vi "setting.vi"() -> ()   [LabVIEW 2019, in "Setting Lib.lvlib"]
uses:
  Setting Lib.lvlib
  User Lib.lvlib
  Calibration Lib.lvlib
  database.lvlib
panel:
  out "Error out 4":errorcluster
  in  "Error in 2":errorcluster
  out "Error out 3":errorcluster
  out "Error out 2":errorcluster
  out "Error out":errorcluster
  out "String":string
  in  "Close":bool
  in  "Calibration":bool
  in  "General":bool
  in  "Speed Control":bool
  in  "User":bool
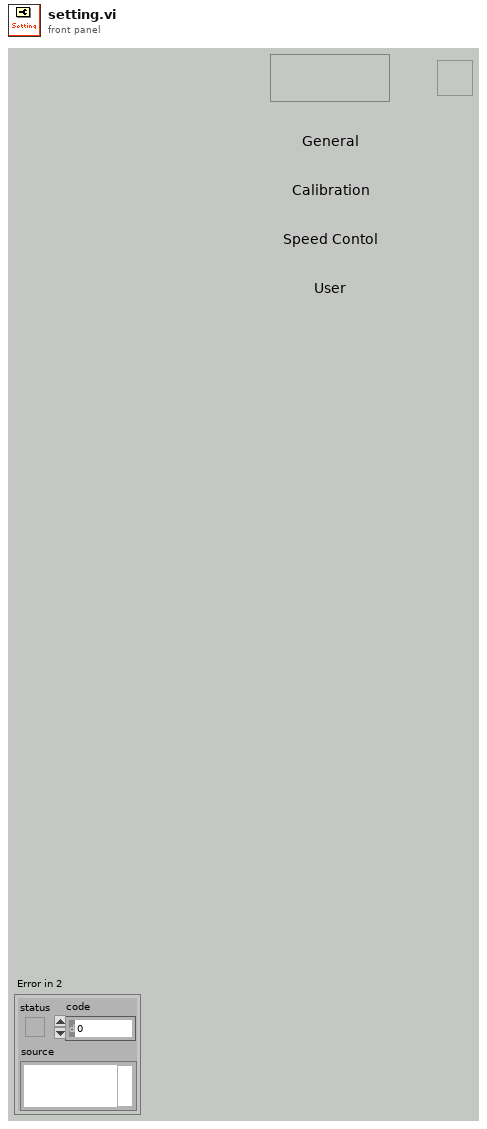
[diagram p1: front panel]
types:
  T1 = cluster{string, "date/time string":string, "date/time string":string, string}
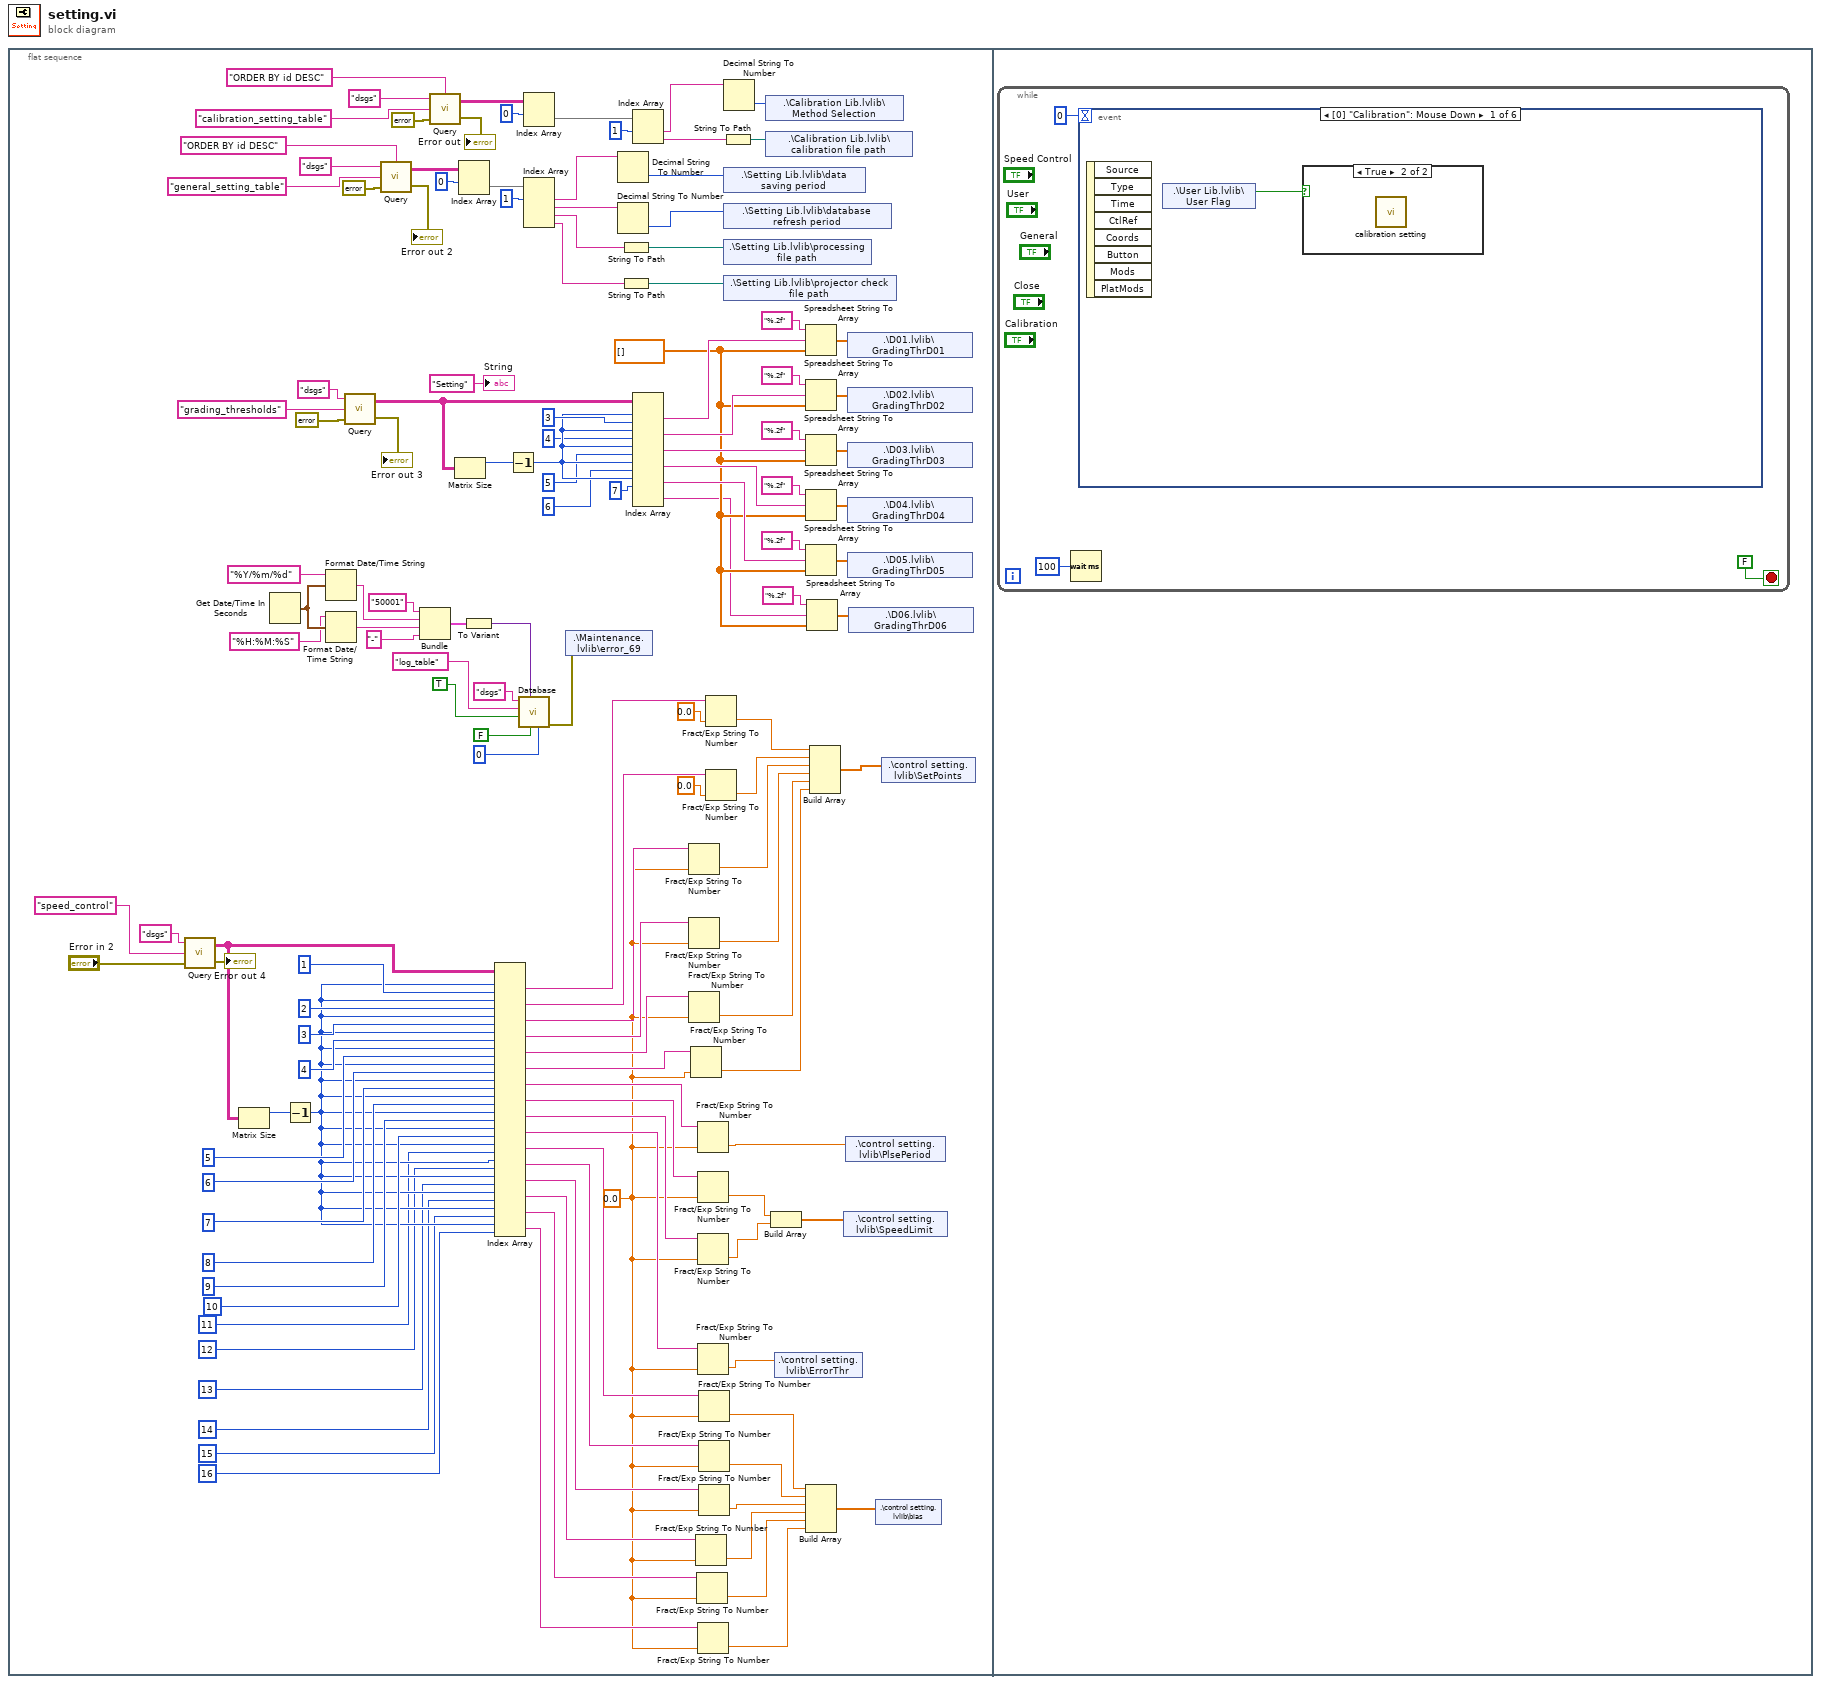
[diagram p0: block diagram]
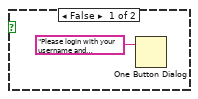
[diagram p2: hidden frame]
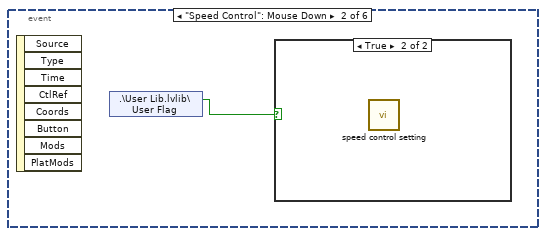
[diagram p3: hidden frame]
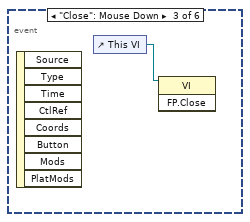
[diagram p5: hidden frame]
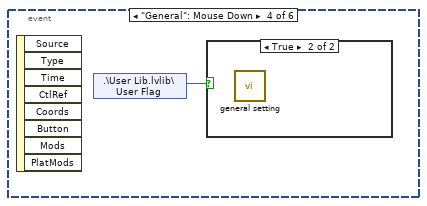
[diagram p6: hidden frame]
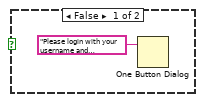
[diagram p7: hidden frame]
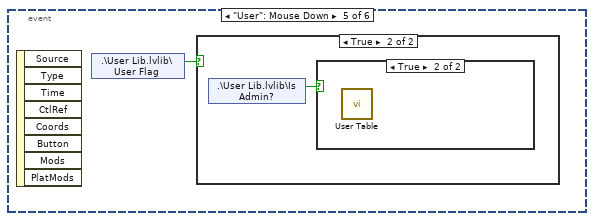
[diagram p8: hidden frame]
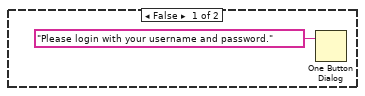
[diagram p9: hidden frame]
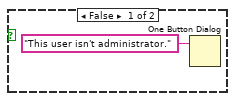
[diagram p10: hidden frame]
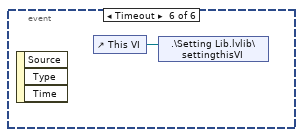
[diagram p11: hidden frame]
diagram:
  n1 = flat-sequence {
    frame #0 {
      w8 = 0.0 ("default (0 DBL)")
      w30 = dbl[] []
      n2 = call "Query.vi"("Error in"="Error in 2", "Table Name"="speed_control", "Connection Name"="dsgs") -> ("Error out"=→"Error out 4":errorcluster, "data"=w45:string[][])  [unwired: 1 in]
      n3 = Matrix Size(0:w45) -> (1:w62:i32)  [unwired: 1 out]
      n4 = Get Date/Time In Seconds() -> (seconds since 1Jan1904=w77:timestamp)
      n5 = Decrement(x=w62) -> (x-1=w21:i32)
      n6 = Format Date/Time String(time format string (%c)="%Y/%m/%d", seconds (now)=w77) -> (date/time string=w74:string)  [unwired: 1 in]
      n7 = Format Date/Time String(time format string (%c)="%H:%M:%S", seconds (now)=w77) -> (date/time string=w73:string)  [unwired: 1 in]
      n8 = call "Query.vi"("Error in"=errorcluster {"status"=FALSE, "code"=0, "source"=""}, "Table Name"="grading_thresholds", "Connection Name"="dsgs") -> ("Error out"=→"Error out 3":errorcluster, "data"=w136:string[][])  [unwired: 1 in]
      n9 = call "Query.vi"("Condition"="ORDER BY id DESC", "Error in"=errorcluster {"status"=FALSE, "code"=0, "source"=""}, "Table Name"="general_setting_table", "Connection Name"="dsgs") -> ("Error out"=→"Error out 2":errorcluster, "data"=w108:string[][])
      n10 = Bundle("50001", "date/time string"=w74, "date/time string"=w73, "-") -> (w71:T1)  [unwired: 1 in]
      n11 = call "Query.vi"("Condition"="ORDER BY id DESC", "Error in"=errorcluster {"status"=FALSE, "code"=0, "source"=""}, "Table Name"="calibration_setting_table", "Connection Name"="dsgs") -> ("Error out"=→"Error out":errorcluster, "data"=w90:string[][])
      n12 = Matrix Size(0:w136) -> (1:w135:i32)  [unwired: 1 out]
      n13 = Index Array(array=w108, index (row)=0) -> (element=w106:string[])  [unwired: 1 in]
      n14 = To Variant(anything=w71) -> (Variant=w70:variant)
      n15 = Index Array(array=w45, index (row) #1=w21, index (col) #1=1 ("disabled index (col)"), index (row) #2=w21, index (col) #2=2 ("disabled index (col)"), index (row) #3=w21, index (col) #3=3 ("disabled index (col)"), index (row) #4=w21, index (col) #4=4 ("disabled index (col)"), index (row) #5=w21, index (col) #5=5 ("disabled index (col)"), index (row) #6=w21, index (col) #6=6 ("disabled index (col)"), index (row) #7=w21, index (col) #7=7 ("disabled index (col)"), index (row) #8=w21, index (col) #8=8 ("disabled index (col)"), index (row) #9=w21, index (col) #9=9 ("disabled index (col)"), index (row) #10=w21, index (col) #10=10 ("disabled index (col)"), index (row) #11=w21, index (col) #11=11 ("disabled index (col)"), index (row) #12=w21, index (col) #12=12 ("disabled index (col)"), index (row) #13=w21, index (col) #13=13 ("disabled index (col)"), index (row) #14=w21, index (col) #14=14 ("disabled index (col)"), index (row) #15=w21, index (col) #15=15 ("disabled index (col)"), index (row) #16=w21, index (col) #16=16 ("disabled index (col)")) -> (element #1=w52:string, element #2=w49:string, element #3=w48:string, element #4=w47:string, element #5=w46:string, element #6=w23:string, element #7=w24:string, element #8=w25:string, element #9=w26:string, element #10=w27:string, element #11=w14:string, element #12=w13:string, element #13=w12:string, element #14=w11:string, element #15=w10:string, element #16=w9:string)
      n16 = Decrement(x=w135) -> (x-1=w133:i32)
      n17 = call "Database.vi"("Maximum Row"=u64 0 ("Storage Time (Day)"), "Delete row?"=FALSE, "Data"=w70, "Auto Increment ID?"=TRUE, "Table"="log_table", "Connection"="dsgs") -> ("Error out"=w66:errorcluster)  [unwired: 5 in]
      n18 = Index Array(array=w90, index (row)=0) -> (element=w92:string[])  [unwired: 1 in]
      n19 = Index Array(array=w106, index #1=1 ("index")) -> (element #1=w104:string, element #2=w103:string, element #3=w102:string, element #4=w101:string)  [unwired: 3 in]
      n20 = shared-variable ".\\Maintenance.lvlib\\error_69"(w66) -> ()  [unwired: 1 in, 1 out]
      n21 = Decimal String To Number(string=w104) -> (number=w97:i32)  [unwired: 2 in, 1 out]
      n22 = Decimal String To Number(string=w103) -> (number=w98:i32)  [unwired: 2 in, 1 out]
      n23 = String To Path(string=w102) -> (path=w99:path)
      n24 = String To Path(string=w101) -> (path=w100:path)
      n25 = Index Array(array=w92, index #1=1 ("index")) -> (element #1=w94:string, element #2=w85:string)  [unwired: 1 in]
      n26 = Index Array(array=w136, index (row) #1=w133, index (col) #1=3 ("disabled index (col)"), index (row) #2=w133, index (col) #2=4 ("disabled index (col)"), index (row) #3=w133, index (col) #3=5 ("disabled index (col)"), index (row) #4=w133, index (col) #4=6 ("disabled index (col)"), index (row) #5=w133, index (col) #5=7 ("disabled index (col)")) -> (element #1=w128:string, element #2=w122:string, element #3=w121:string, element #4=w120:string, element #5=w119:string, element #6=w29:string)  [unwired: 2 in]
      n27 = Fract/Exp String To Number(string=w48, default (0 dbl)=w8) -> (number=w42:dbl)  [unwired: 2 in, 1 out]
      n28 = Fract/Exp String To Number(string=w47, default (0 dbl)=w8) -> (number=w41:dbl)  [unwired: 2 in, 1 out]
      n29 = Fract/Exp String To Number(string=w46, default (0 dbl)=w8) -> (number=w40:dbl)  [unwired: 2 in, 1 out]
      n30 = Fract/Exp String To Number(string=w23, default (0 dbl)=w8) -> (number=w22:dbl)  [unwired: 2 in, 1 out]
      n31 = Fract/Exp String To Number(string=w11, default (0 dbl)=w8) -> (number=w4:dbl)  [unwired: 2 in, 1 out]
      n32 = Fract/Exp String To Number(string=w10, default (0 dbl)=w8) -> (number=w3:dbl)  [unwired: 2 in, 1 out]
      n33 = Fract/Exp String To Number(string=w24, default (0 dbl)=w8) -> (number=w38:dbl)  [unwired: 2 in, 1 out]
      n34 = Fract/Exp String To Number(string=w25, default (0 dbl)=w8) -> (number=w37:dbl)  [unwired: 2 in, 1 out]
      n35 = Fract/Exp String To Number(string=w26, default (0 dbl)=w8) -> (number=w36:dbl)  [unwired: 2 in, 1 out]
      n36 = Fract/Exp String To Number(string=w27, default (0 dbl)=w8) -> (number=w34:dbl)  [unwired: 2 in, 1 out]
      n37 = Fract/Exp String To Number(string=w9, default (0 dbl)=w8) -> (number=w2:dbl)  [unwired: 2 in, 1 out]
      n38 = Fract/Exp String To Number(string=w14, default (0 dbl)=w8) -> (number=w7:dbl)  [unwired: 2 in, 1 out]
      n39 = Fract/Exp String To Number(string=w13, default (0 dbl)=w8) -> (number=w6:dbl)  [unwired: 2 in, 1 out]
      n40 = Fract/Exp String To Number(string=w12, default (0 dbl)=w8) -> (number=w5:dbl)  [unwired: 2 in, 1 out]
      n41 = Fract/Exp String To Number(string=w52, default (0 dbl)=0.0 ("default (0 DBL)")) -> (number=w44:dbl)  [unwired: 2 in, 1 out]
      n42 = Fract/Exp String To Number(string=w49, default (0 dbl)=0.0 ("default (0 DBL)")) -> (number=w43:dbl)  [unwired: 2 in, 1 out]
      n43 = String To Path(string=w85) -> (path=w95:path)
      n44 = Decimal String To Number(string=w94) -> (number=w96:i32)  [unwired: 2 in, 1 out]
      n45 = shared-variable ".\\Setting Lib.lvlib\\data saving period"(w97) -> ()  [unwired: 1 in, 1 out]
      n46 = shared-variable ".\\Setting Lib.lvlib\\database refresh period"(w98) -> ()  [unwired: 1 in, 1 out]
      n47 = shared-variable ".\\Setting Lib.lvlib\\processing file path"(w99) -> ()  [unwired: 1 in, 1 out]
      n48 = shared-variable ".\\Setting Lib.lvlib\\projector check file path"(w100) -> ()  [unwired: 1 in, 1 out]
      n49 = shared-variable ".\\Calibration Lib.lvlib\\Method Selection"(w96) -> ()  [unwired: 1 in, 1 out]
      n50 = shared-variable ".\\Calibration Lib.lvlib\\calibration file path"(w95) -> ()  [unwired: 1 in, 1 out]
      n51 = Build Array(w37, w36) -> (w35:dbl[])
      n52 = shared-variable ".\\control setting.lvlib\\ErrorThr"(w34) -> ()  [unwired: 1 in, 1 out]
      n53 = Spreadsheet String To Array(format string="%.2f", spreadsheet string=w128, array type (2D Dbl)=w30) -> (array=w118:dbl[])  [unwired: 1 in]
      n54 = Spreadsheet String To Array(format string="%.2f", spreadsheet string=w122, array type (2D Dbl)=w30) -> (array=w117:dbl[])  [unwired: 1 in]
      n55 = Spreadsheet String To Array(format string="%.2f", spreadsheet string=w121, array type (2D Dbl)=w30) -> (array=w116:dbl[])  [unwired: 1 in]
      n56 = Spreadsheet String To Array(format string="%.2f", spreadsheet string=w120, array type (2D Dbl)=w30) -> (array=w115:dbl[])  [unwired: 1 in]
      n57 = Spreadsheet String To Array(format string="%.2f", spreadsheet string=w119, array type (2D Dbl)=w30) -> (array=w114:dbl[])  [unwired: 1 in]
      n58 = Build Array(w7, w6, w5, w4, w3, w2) -> (w1:dbl[])
      n59 = Spreadsheet String To Array(format string="%.2f", spreadsheet string=w29, array type (2D Dbl)=w30) -> (array=w32:dbl[])  [unwired: 1 in]
      n60 = Build Array(w44, w43, w42, w41, w40, w22) -> (w39:dbl[])
      n61 = shared-variable ".\\control setting.lvlib\\SpeedLimit"(w35) -> ()  [unwired: 1 in, 1 out]
      n62 = shared-variable ".\\control setting.lvlib\\PlsePeriod"(w38) -> ()  [unwired: 1 in, 1 out]
      n63 = shared-variable ".\\D01.lvlib\\GradingThrD01"(w118) -> ()  [unwired: 1 in, 1 out]
      n64 = shared-variable ".\\D02.lvlib\\GradingThrD02"(w117) -> ()  [unwired: 1 in, 1 out]
      n65 = shared-variable ".\\D03.lvlib\\GradingThrD03"(w116) -> ()  [unwired: 1 in, 1 out]
      n66 = shared-variable ".\\D04.lvlib\\GradingThrD04"(w115) -> ()  [unwired: 1 in, 1 out]
      n67 = shared-variable ".\\D05.lvlib\\GradingThrD05"(w114) -> ()  [unwired: 1 in, 1 out]
      n68 = shared-variable ".\\D06.lvlib\\GradingThrD06"(w32) -> ()  [unwired: 1 in, 1 out]
      n69 = shared-variable ".\\control setting.lvlib\\bias"(w1) -> ()  [unwired: 1 in, 1 out]
      n70 = shared-variable ".\\control setting.lvlib\\SetPoints"(w39) -> ()  [unwired: 1 in, 1 out]
      "String" <- "Setting" ("String")
    }
    frame #1 {
      n71 = while {
        stop <- FALSE stop-if-true
        n72 = Wait (ms)(milliseconds to wait=u32 100) -> ()  [unwired: 1 out]
        n73 = event shown="[0] \"Calibration\": Mouse Down" {
          selector: _ -> [_ _ _ _ _ _]
          dyn-events: _ -> [_ _ _ _ _ _]
          timeout: 0 -> [_ _ _ _ _ _]
          event "Calibration": Mouse Down {
            n74 = event-data() -> ()  [unwired: 1 in, 8 out]
            n75 = shared-variable ".\\User Lib.lvlib\\User Flag"() -> (w142:bool)  [unwired: 1 in, 1 out]
            n76 = case shown="True" w142 {
              frame False {
                n77 = One Button Dialog(message="Please login with your username and password.") -> ()  [unwired: 1 in, 1 out]
              }
              frame True {
                n78 = call "calibration setting.vi"() -> ()  [unwired: 12 in]
              }
            }
          }
          event "Speed Control": Mouse Down {
            n79 = event-data() -> ()  [unwired: 1 in, 8 out]
            n80 = shared-variable ".\\User Lib.lvlib\\User Flag"() -> (w144:bool)  [unwired: 1 in, 1 out]
            n81 = case shown="True" w144 {
              frame False {
              }
              frame True {
                n82 = call "speed control setting.vi"() -> ()  [unwired: 12 in]
              }
            }
          }
          event "Close": Mouse Down {
            n83 = event-data() -> ()  [unwired: 1 in, 8 out]
            n84 = control-ref of="This VI"() -> (w145:refnum<vi>)
            n85 = invoke class="VI" method="FP.Close"(reference=w145) -> ()  [unwired: 2 in, 3 out]
          }
          event "General": Mouse Down {
            n86 = event-data() -> ()  [unwired: 1 in, 8 out]
            n87 = shared-variable ".\\User Lib.lvlib\\User Flag"() -> (w146:bool)  [unwired: 1 in, 1 out]
            n88 = case shown="True" w146 {
              frame False {
                n89 = One Button Dialog(message="Please login with your username and password.") -> ()  [unwired: 1 in, 1 out]
              }
              frame True {
                n90 = call "general setting.vi"() -> ()  [unwired: 12 in]
              }
            }
          }
          event "User": Mouse Down {
            n91 = event-data() -> ()  [unwired: 1 in, 8 out]
            n92 = shared-variable ".\\User Lib.lvlib\\User Flag"() -> (w148:bool)  [unwired: 1 in, 1 out]
            n93 = case shown="True" w148 {
              frame False {
                n94 = One Button Dialog(message="Please login with your username and password.") -> ()  [unwired: 1 in, 1 out]
              }
              frame True {
                n95 = shared-variable ".\\User Lib.lvlib\\Is Admin?"() -> (w150:bool)  [unwired: 1 in, 1 out]
                n96 = case shown="True" w150 {
                  frame False {
                    n97 = One Button Dialog(message="This user isn't administrator.") -> ()  [unwired: 1 in, 1 out]
                  }
                  frame True {
                    n98 = call "User Table.vi"() -> ()  [unwired: 12 in]
                  }
                }
              }
            }
          }
          event Timeout {
            n99 = event-data() -> ()  [unwired: 1 in, 3 out]
            n100 = control-ref of="This VI"() -> (w152:refnum<vi>)
            n101 = shared-variable ".\\Setting Lib.lvlib\\settingthisVI"(w152) -> ()  [unwired: 1 in, 1 out]
          }
        }
      }
    }
  }
